vi "Outcome - When Not Set Explicitly - Is None.vi"() -> ()   [LabVIEW 2017, in "Test Result.Tests.lvlib"]
uses:
  Test Result.Tests.lvlib
  Test Result/Test Result.lvclass
  Test Result/Test Result.lvclass/Test Result.ctl
  Test Outcome.ctl
  605ee93e-48c1-4eff-9957-e73fe43c526f.vi
  Test Result/Get Outcome.vi
  <vilib>/PNR/Transparent Assertions/Transparent Assertions/Constraints/IsEqual/Create.vi
  <vilib>/PNR/Transparent Assertions/Transparent Assertions/Constraints/IsEqual/IsEqual.lvclass
panel:
  out "error out":errorcluster
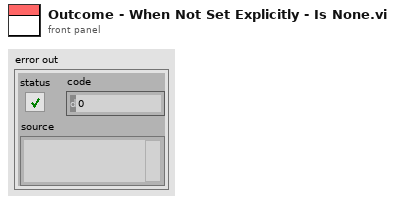
[diagram p1: front panel]
types:
  T1 = typedef "Test Outcome.ctl" = enum16{"None", "Passed", "Failed"}
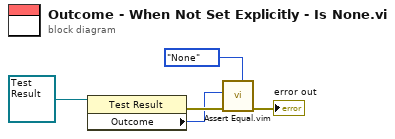
[diagram p0: block diagram]
diagram:
  n1 = property class="Test Result"(reference=refnum<class "Test Result.lvclass"> refnum ("Test Result")) -> (error out=w4:errorcluster, "Outcome"=w3:T1)  [unwired: 1 in, 1 out]
  n2 = call "Assert Equal.vim"("Expected"=Test_Outcome."None" ("Test Outcome"), "error in (no error)"=w4, "Actual"=w3) -> ("error out"=→"error out":errorcluster)  [unwired: 8 in]
